vi "4461 - Create IO Channels Parallel.vi"(6 "error in":errorcluster, 7 "AI Buffer Size (S)":i32=10, 8 "sampling info":cluster{"Fs":dbl, "#s":dbl}, 9 "AO":T1={"AO amp (V)"=[0.1, 0.09, 0.08, 0.07, 0.06, 0.05, 0.04, 0.03], "AO DC (V)"=[0.0, 0.0, 0.0, 0.0, 0.0, 0.0, 0.0, 0.0], "AO f (Hz)"=[13.0, 13.0, 13.0, 13.0, 13.0, 13.0, 13.0, 13.0], "AO phi (deg)"=[0.0, 0.0, 0.0, 0.0, 0.0, 0.0, 0.0, 0.0], "function"=[enum."Sine Wave", enum."Sine Wave", enum."Sine Wave", enum."Sine Wave", enum."Sine Wave", enum."Sine Wave", enum."Sine Wave", enum."Sine Wave"]} {"AO DC (V)" format="%#_6p"; "AO amp (V)" format="%#_6p"}, 10 "AO Configuration":T2(array[cluster])=[{"Output physical channels"="PXI1Slot2/ao0", "AO. Max"=0.1, "AO.Min"=-0.1}, {"Output physical channels"="", "AO. Max"=0.1, "AO.Min"=-0.1}], 11 "AI Configuration":T3(array[cluster])=[{"AI.Coupling"=10050, "AI.Max"=10.0, "AI.Min"=-10.0, "Input physical channels"="PXI1Slot2/ai0:1"}, {"AI.Coupling"=10050, "AI.Max"=10.0, "AI.Min"=-10.0, "Input physical channels"="PXI1Slot3/ai0:3"}, {"AI.Coupling"=10050, "AI.Max"=10.0, "AI.Min"=-10.0, "Input physical channels"=""}] {"AI.Coupling" items=["AC"=10045, "DC"=10050, "GND"=10066]}) -> (2 "AO Task":refnum<k21>[](array[refnum]), 3 "AI task":refnum<k21>[](array[refnum]), 4 "error out":errorcluster, 5 "phase log":dbl[](array[numeric])=[0.99999999999938, 0.99999999999938])   [LabVIEW 2013]
uses:
  <vilib>/DAQmx/write.llb/DAQmx Write (Analog 1D Wfm NChan NSamp).vi
  <vilib>/DAQmx/create/channels.llb/DAQmx Create Channel (AO-Voltage-Basic).vi
  <vilib>/DAQmx/create/channels.llb/DAQmx Create Channel (AI-Voltage-Basic).vi
  <vilib>/DAQmx/configure/timing.llb/DAQmx Timing (Sample Clock).vi
  <vilib>/DAQmx/configure/trigger.llb/DAQmx Start Trigger (Digital Edge).vi
  <vilib>/DAQmx/miscellaneous.llb/DAQmx Fill In Error Info.vi
  <resource>/objmgr/daqmx.rc
panel:
  out "AI.FilterDelay":dbl
  out "AI.Gain":dbl
  in  "input terminal configuration":i32(ring)=-1 items=["default"=-1, "RSE"=10083, "NRSE"=10078, "Differential"=10106, "Pseudodifferential"=12529]
  in  "output terminal configuration":i32(ring)=-1 items=["Default"=-1, "RSE"=10083, "Differential"=10106, "Pseudodifferential"=12529]
  out "SampClk.Timebase.Rate":dbl
  out "SampQuant.SampPerChan":dbl
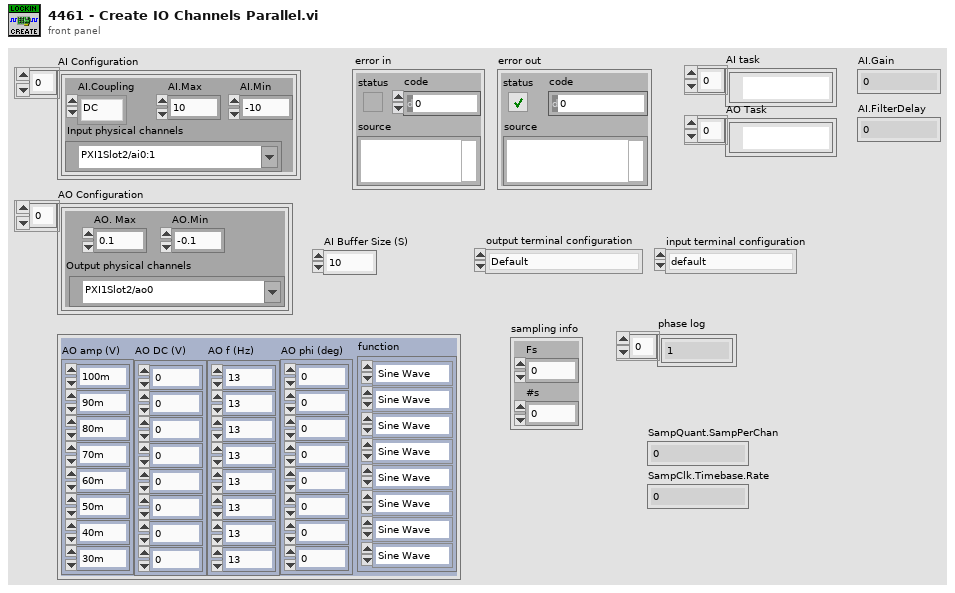
[diagram p1: front panel]
types:
  T1 = cluster{"AO amp (V)":dbl[], "AO DC (V)":dbl[], "AO f (Hz)":dbl[], "AO phi (deg)":dbl[], "function":enum16{"Sine Wave", "Triangle Wave", "Square Wave", "Sawtooth Wave"}[]}
  T2 = cluster{"Output physical channels":tag, "AO. Max":dbl, "AO.Min":dbl}[]
  T3 = cluster{"AI.Coupling":i32, "AI.Max":dbl, "AI.Min":dbl, "Input physical channels":tag}[]
  T4 = cluster{"AI.Coupling":i32, "AI.Max":dbl, "AI.Min":dbl, "Input physical channels":tag}
  T5 = cluster{"Output physical channels":tag, "AO. Max":dbl, "AO.Min":dbl}
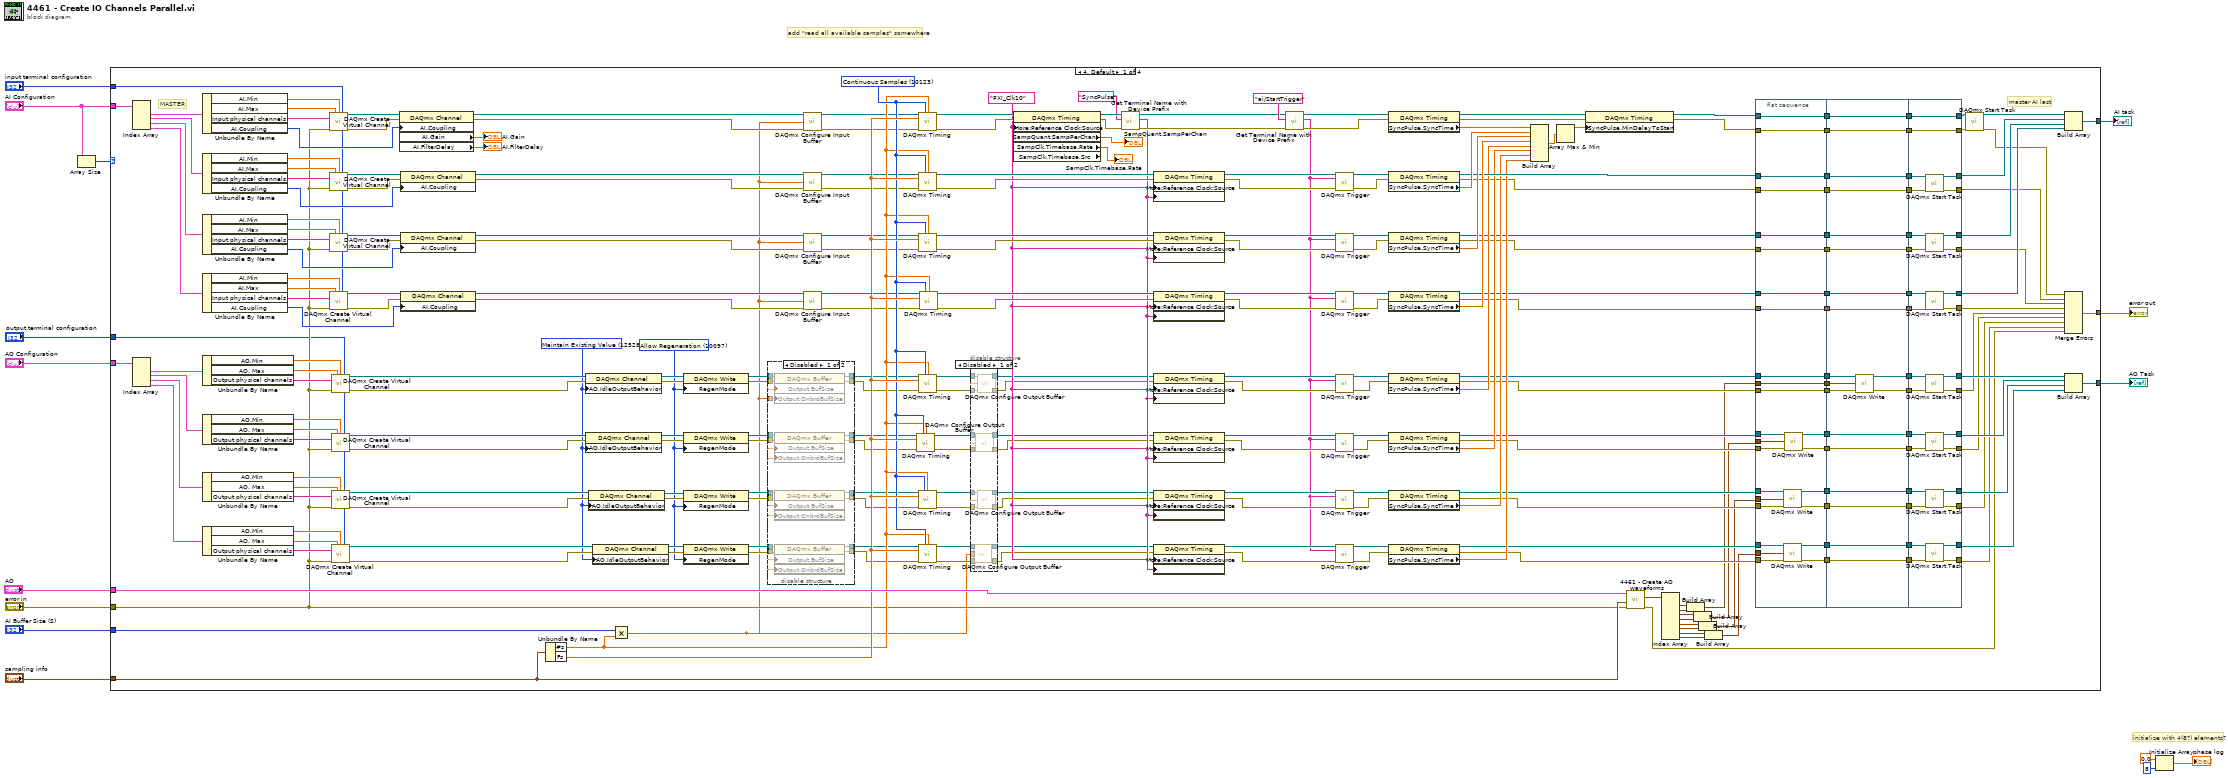
[diagram p0: block diagram]
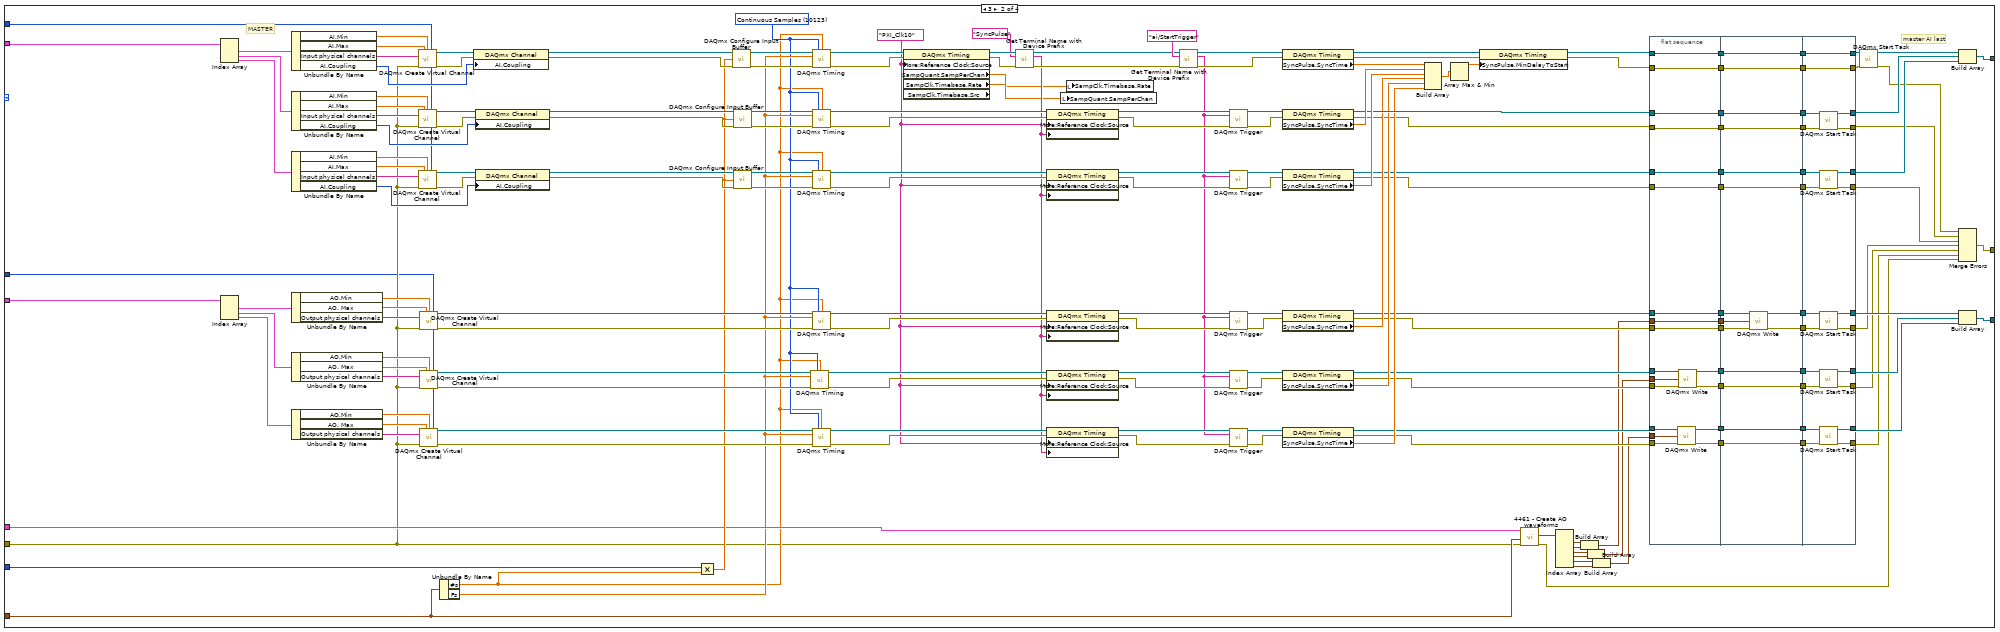
[diagram p4: hidden frame]
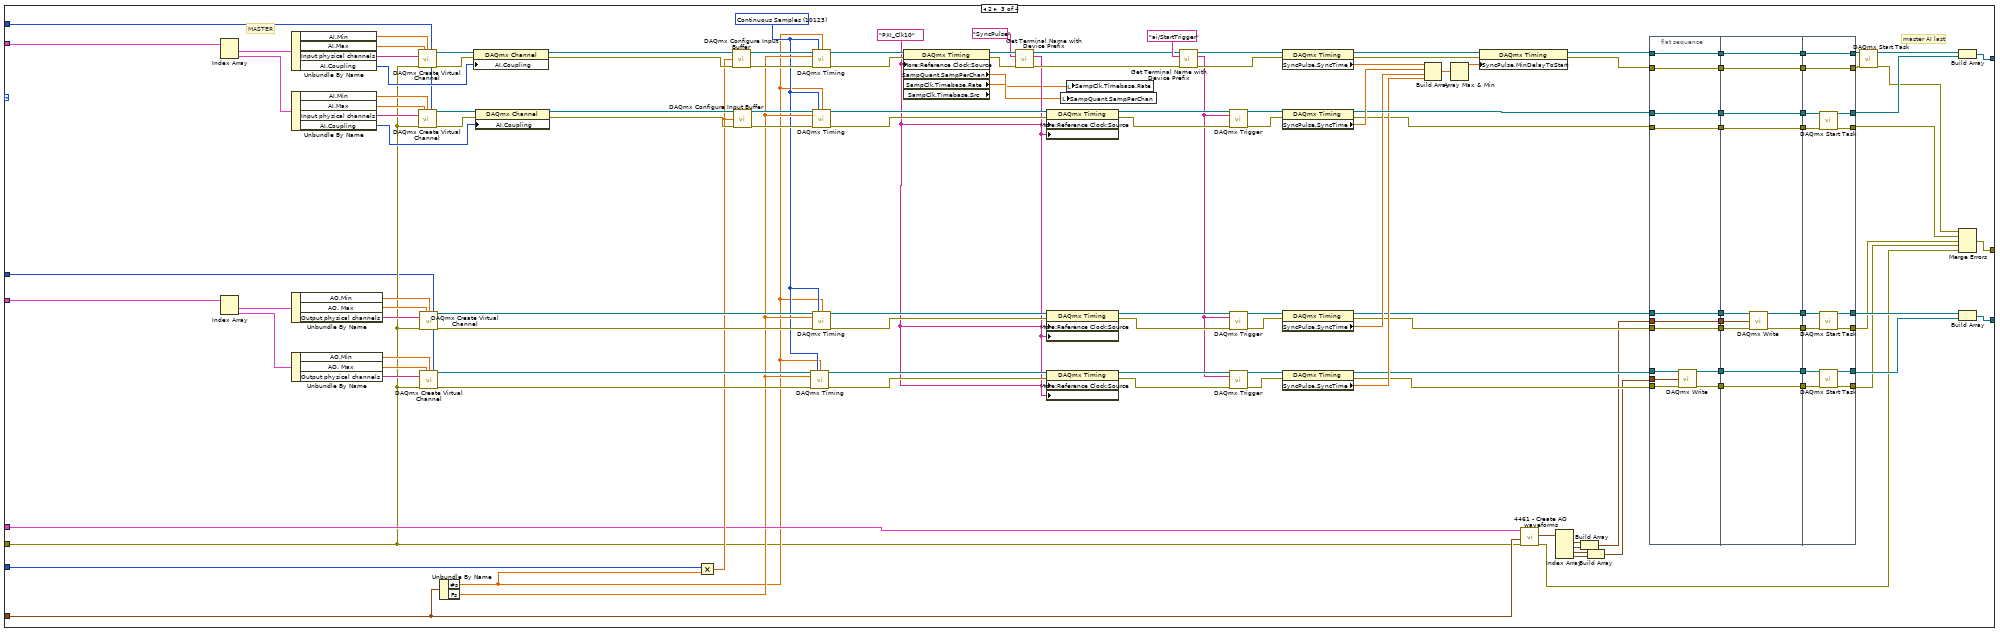
[diagram p5: hidden frame]
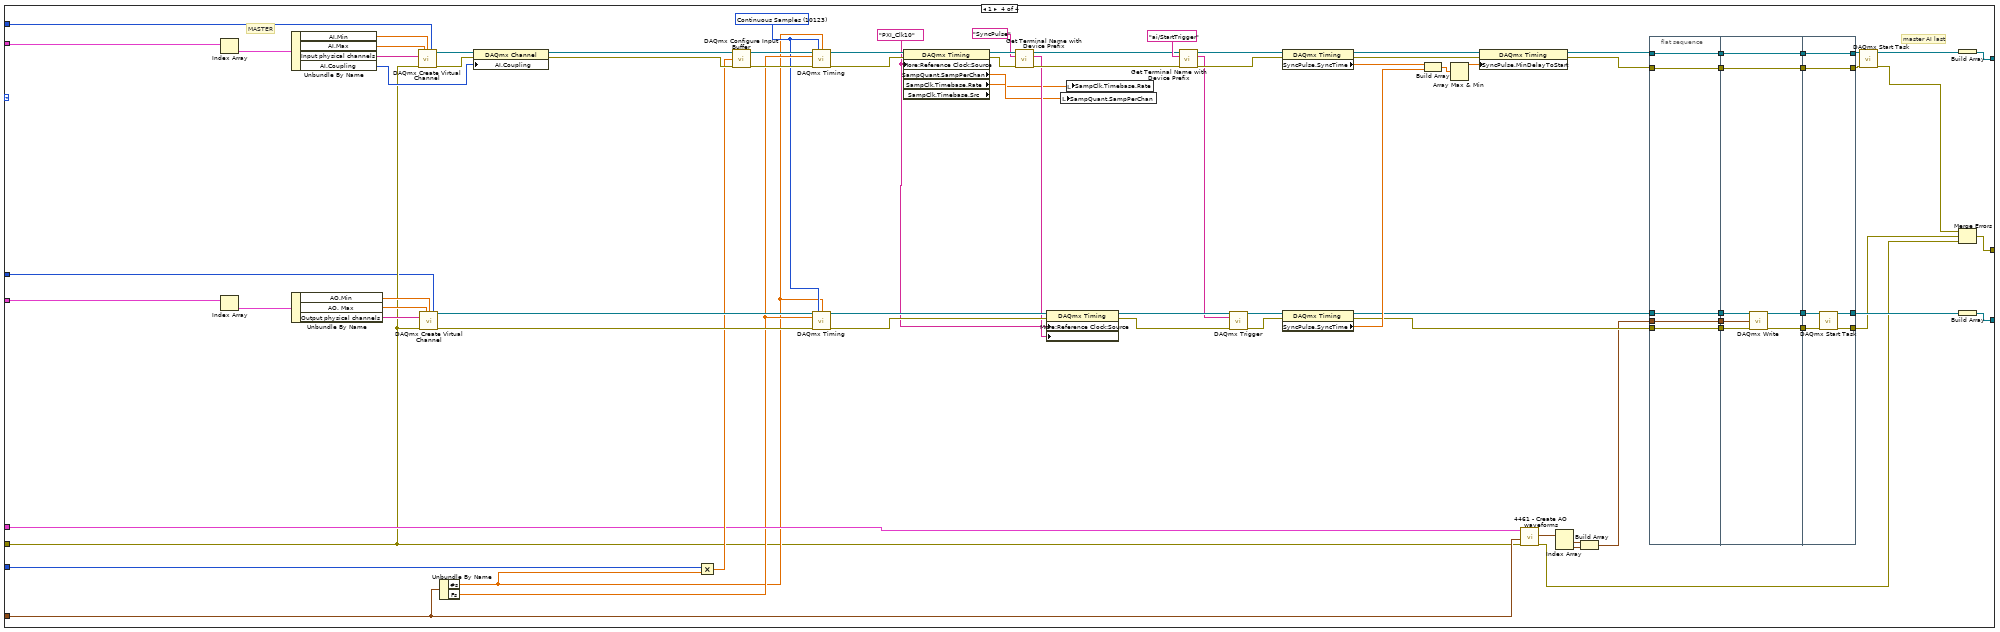
[diagram p6: hidden frame]
diagram:
  # "initialize with 4(8?) elements?"
  # "add \"read all available samples\" somewhere"
  n1 = Array Size(array="AI Configuration") -> (size(s)=w3:i32)
  n2 = case shown="4, Default" w3 {
    tunnel: "AI Buffer Size (S)" -> [w233 w545 w742 w870]
    tunnel: [w231 w543 w740 w868] -> w14
    tunnel: "AI Configuration" -> [w230 w542 w739 w867]
    tunnel: "AO Configuration" -> [w181 w499 w714 w861]
    tunnel: [w123 w446 w680 w845] -> w12
    tunnel: "AO" -> [w105 w428 w665 w833]
    tunnel: "sampling info" -> [w104 w427 w664 w832]
    tunnel: [w96 w420 w658 w827] -> w6
    tunnel: "error in" -> [w90 w415 w654 w824]
    tunnel: "output terminal configuration" -> [w85 w410 w650 w819]
    tunnel: "input terminal configuration" -> [w86 w411 w649 w820]
    frame 4, Default {
      w74 = 12528 items=["Zero Volts"=12526, "High-Impedance"=12527, "Maintain Existing Value"=12528] ("AO.IdleOutputBehavior")
      w49 = 10097 items=["Allow Regeneration"=10097, "Do Not Allow Regeneration"=10158] ("RegenMode")
      w118 = tag "PXI_Clk10" ("RefClk.Src")
      w102 = 10123 items=["Finite Samples"=10178, "Continuous Samples"=10123] ("sample mode")
      # "master AI last"
      # "MASTER"
      n3 = Index Array(array=w230) -> (element #1=w251:T4, element #2=w219:T4, element #3=w194:T4, element #4=w193:T4)  [unwired: 4 in]
      n4 = Index Array(array=w181) -> (element #1=w180:T5, element #2=w149:T5, element #3=w150:T5, element #4=w151:T5)  [unwired: 4 in]
      n5 = Unbundle By Name(w251) -> ("AI.Min"=w228:dbl, "AI.Max"=w229:dbl, "Input physical channels"=w236:tag, "AI.Coupling"=w227:i32)
      n6 = Unbundle By Name(w219) -> ("AI.Min"=w224:dbl, "AI.Max"=w223:dbl, "Input physical channels"=w220:tag, "AI.Coupling"=w225:i32)
      n7 = Unbundle By Name(w194) -> ("AI.Min"=w206:dbl, "AI.Max"=w207:dbl, "Input physical channels"=w210:tag, "AI.Coupling"=w205:i32)
      n8 = Unbundle By Name(w193) -> ("AI.Min"=w203:dbl, "AI.Max"=w202:dbl, "Input physical channels"=w199:tag, "AI.Coupling"=w204:i32)
      n9 = Unbundle By Name(w180) -> ("AO.Min"=w177:dbl, "AO. Max"=w178:dbl, "Output physical channels"=w179:tag)
      n10 = Unbundle By Name(w149) -> ("AO.Min"=w168:dbl, "AO. Max"=w167:dbl, "Output physical channels"=w166:tag)
      n11 = Unbundle By Name(w150) -> ("AO.Min"=w163:dbl, "AO. Max"=w164:dbl, "Output physical channels"=w165:tag)
      n12 = Unbundle By Name(w151) -> ("AO.Min"=w154:dbl, "AO. Max"=w153:dbl, "Output physical channels"=w152:tag)
      n13 = call-poly <vilib>:"DAQmx Create Virtual Channel.vi"("maximum value"=w229, "minimum value"=w228, "input terminal configuration"=w86, "physical channels"=w236, "error in"=w90) -> ("task out"=w235:refnum<k21>, "error out"=w234:errorcluster)  [unwired: 9 in]
      n14 = call-poly <vilib>:"DAQmx Create Virtual Channel.vi"("maximum value"=w223, "minimum value"=w224, "input terminal configuration"=w86, "physical channels"=w220, "error in"=w90) -> ("task out"=w221:refnum<k21>, "error out"=w222:errorcluster)  [unwired: 9 in]
      n15 = call-poly <vilib>:"DAQmx Create Virtual Channel.vi"("maximum value"=w207, "minimum value"=w206, "input terminal configuration"=w86, "physical channels"=w210, "error in"=w90) -> ("task out"=w209:refnum<k21>, "error out"=w208:errorcluster)  [unwired: 9 in]
      n16 = call-poly <vilib>:"DAQmx Create Virtual Channel.vi"("maximum value"=w202, "minimum value"=w203, "input terminal configuration"=w86, "physical channels"=w199, "error in"=w90) -> ("task out"=w200:refnum<k21>, "error out"=w201:errorcluster)  [unwired: 9 in]
      n17 = call-poly <vilib>:"DAQmx Create Virtual Channel.vi"("maximum value"=w178, "minimum value"=w177, "output terminal configuration"=w85, "physical channels"=w179, "error in"=w90) -> ("task out"=w82:refnum<k21>, "error out"=w81:errorcluster)  [unwired: 9 in]
      n18 = call-poly <vilib>:"DAQmx Create Virtual Channel.vi"("maximum value"=w167, "minimum value"=w168, "output terminal configuration"=w85, "physical channels"=w166, "error in"=w90) -> ("task out"=w75:refnum<k21>, "error out"=w76:errorcluster)  [unwired: 9 in]
      n19 = call-poly <vilib>:"DAQmx Create Virtual Channel.vi"("maximum value"=w164, "minimum value"=w163, "output terminal configuration"=w85, "physical channels"=w165, "error in"=w90) -> ("task out"=w77:refnum<k21>, "error out"=w78:errorcluster)  [unwired: 9 in]
      n20 = call-poly <vilib>:"DAQmx Create Virtual Channel.vi"("maximum value"=w153, "minimum value"=w154, "output terminal configuration"=w85, "physical channels"=w152, "error in"=w90) -> ("task out"=w80:refnum<k21>, "error out"=w79:errorcluster)  [unwired: 9 in]
      n21 = property class="DAQmx Channel"(reference=w235, error in=w234, "AI.Coupling"=w227) -> (reference out=w32:refnum<k21>, error out=w20:errorcluster, "AI.Gain"=→"AI.Gain":dbl, "AI.FilterDelay"=→"AI.FilterDelay":dbl)
      n22 = property class="DAQmx Channel"(reference=w221, error in=w222, "AI.Coupling"=w225) -> (reference out=w30:refnum<k21>, error out=w19:errorcluster)
      n23 = property class="DAQmx Channel"(reference=w209, error in=w208, "AI.Coupling"=w205) -> (reference out=w29:refnum<k21>, error out=w18:errorcluster)
      n24 = property class="DAQmx Channel"(reference=w200, error in=w201, "AI.Coupling"=w204) -> (reference out=w28:refnum<k21>, error out=w17:errorcluster)
      n25 = Unbundle By Name(w104) -> ("#s"=w101:dbl, "Fs"=w103:dbl)
      n26 = property class="DAQmx Channel"(reference=w82, error in=w81, "AO.IdleOutputBehavior"=w74) -> (reference out=w65:refnum<k21>, error out=w64:errorcluster)
      n27 = property class="DAQmx Channel"(reference=w75, error in=w76, "AO.IdleOutputBehavior"=w74) -> (reference out=w54:refnum<k21>, error out=w55:errorcluster)
      n28 = property class="DAQmx Channel"(reference=w77, error in=w78, "AO.IdleOutputBehavior"=w74) -> (reference out=w56:refnum<k21>, error out=w57:errorcluster)
      n29 = property class="DAQmx Channel"(reference=w80, error in=w79, "AO.IdleOutputBehavior"=w74) -> (reference out=w61:refnum<k21>, error out=w58:errorcluster)
      n30 = Multiply(x=w233, y=w101) -> (x*y=w16:dbl)
      n31 = property class="DAQmx Write"(reference=w65, error in=w64, "RegenMode"=w49) -> (reference out=w62:refnum<k21>, error out=w63:errorcluster)
      n32 = property class="DAQmx Write"(reference=w54, error in=w55, "RegenMode"=w49) -> (reference out=w53:refnum<k21>, error out=w52:errorcluster)
      n33 = property class="DAQmx Write"(reference=w56, error in=w57, "RegenMode"=w49) -> (reference out=w51:refnum<k21>, error out=w50:errorcluster)
      n34 = property class="DAQmx Write"(reference=w61, error in=w58, "RegenMode"=w49) -> (reference out=w60:refnum<k21>, error out=w59:errorcluster)
      n35 = disable-structure shown="Disabled" {
        disable-tunnel: [w326 w334] -> w73
        disable-tunnel: [w325 w332] -> w72
        disable-tunnel: [w324 w331] -> w71
        disable-tunnel: [w323 w333] -> w70
        disable-tunnel: [w322 w330] -> w69
        disable-tunnel: [w321 w329] -> w68
        disable-tunnel: [w320 w328] -> w67
        disable-tunnel: [w319 w327] -> w66
        disable-tunnel: w63 -> [w318 w333]
        disable-tunnel: w62 -> [w317 w334]
        disable-tunnel: w60 -> [w316 w328]
        disable-tunnel: w59 -> [w315 w327]
        disable-tunnel: w53 -> [w314 w332]
        disable-tunnel: w52 -> [w313 w331]
        disable-tunnel: w51 -> [w312 w330]
        disable-tunnel: w50 -> [w311 w329]
        disable-tunnel: w16 -> [w310 _]
        frame Disabled {
          n36 = property class="DAQmx Buffer"(reference=w317, error in=w318, "Output.BufSize"=w310, "Output.OnbrdBufSize"=w310) -> (reference out=w326:refnum<k21>, error out=w323:errorcluster)
          n37 = property class="DAQmx Buffer"(reference=w314, error in=w313, "Output.BufSize"=w310, "Output.OnbrdBufSize"=w310) -> (reference out=w325:refnum<k21>, error out=w324:errorcluster)
          n38 = property class="DAQmx Buffer"(reference=w312, error in=w311, "Output.BufSize"=w310, "Output.OnbrdBufSize"=w310) -> (reference out=w322:refnum<k21>, error out=w321:errorcluster)
          n39 = property class="DAQmx Buffer"(reference=w316, error in=w315, "Output.BufSize"=w310, "Output.OnbrdBufSize"=w310) -> (reference out=w320:refnum<k21>, error out=w319:errorcluster)
        }
        frame Enabled {
        }
      }
      n40 = call <vilib>:"DAQmx Configure Input Buffer.vi"("task/channels in"=w32, "buffer size (in samples per channel)"=w16, "error in"=w20) -> ("task out"=w31:refnum<k21>, "error out"=w21:errorcluster)  [unwired: 11 in]
      n41 = call <vilib>:"DAQmx Configure Input Buffer.vi"("task/channels in"=w30, "buffer size (in samples per channel)"=w16, "error in"=w19) -> ("task out"=w22:refnum<k21>, "error out"=w23:errorcluster)  [unwired: 11 in]
      n42 = call <vilib>:"DAQmx Configure Input Buffer.vi"("task/channels in"=w29, "buffer size (in samples per channel)"=w16, "error in"=w18) -> ("task out"=w26:refnum<k21>, "error out"=w25:errorcluster)  [unwired: 11 in]
      n43 = call <vilib>:"DAQmx Configure Input Buffer.vi"("task/channels in"=w28, "buffer size (in samples per channel)"=w16, "error in"=w17) -> ("task out"=w27:refnum<k21>, "error out"=w24:errorcluster)  [unwired: 11 in]
      n44 = call-poly <vilib>:"DAQmx Timing.vi"("task/channels in"=w72, "sample mode"=w102, "samples per channel"=w101, "rate"=w103, "error in"=w71) -> ("task out"=w48:refnum<k21>, "error out"=w47:errorcluster)  [unwired: 9 in]
      n45 = call-poly <vilib>:"DAQmx Timing.vi"("task/channels in"=w69, "sample mode"=w102, "samples per channel"=w101, "rate"=w103, "error in"=w68) -> ("task out"=w44:refnum<k21>, "error out"=w41:errorcluster)  [unwired: 9 in]
      n46 = call-poly <vilib>:"DAQmx Timing.vi"("task/channels in"=w31, "sample mode"=w102, "samples per channel"=w101, "rate"=w103, "error in"=w21) -> ("task out"=w250:refnum<k21>, "error out"=w226:errorcluster)  [unwired: 9 in]
      n47 = call-poly <vilib>:"DAQmx Timing.vi"("task/channels in"=w22, "sample mode"=w102, "samples per channel"=w101, "rate"=w103, "error in"=w23) -> ("task out"=w218:refnum<k21>, "error out"=w217:errorcluster)  [unwired: 9 in]
      n48 = call-poly <vilib>:"DAQmx Timing.vi"("task/channels in"=w26, "sample mode"=w102, "samples per channel"=w101, "rate"=w103, "error in"=w25) -> ("task out"=w211:refnum<k21>, "error out"=w212:errorcluster)  [unwired: 9 in]
      n49 = call-poly <vilib>:"DAQmx Timing.vi"("task/channels in"=w73, "sample mode"=w102, "samples per channel"=w101, "rate"=w103, "error in"=w70) -> ("task out"=w34:refnum<k21>, "error out"=w36:errorcluster)  [unwired: 9 in]
      n50 = call-poly <vilib>:"DAQmx Timing.vi"("task/channels in"=w67, "sample mode"=w102, "samples per channel"=w101, "rate"=w103, "error in"=w66) -> ("task out"=w43:refnum<k21>, "error out"=w42:errorcluster)  [unwired: 9 in]
      n51 = call-poly <vilib>:"DAQmx Timing.vi"("task/channels in"=w27, "sample mode"=w102, "samples per channel"=w101, "rate"=w103, "error in"=w24) -> ("task out"=w198:refnum<k21>, "error out"=w197:errorcluster)  [unwired: 9 in]
      n52 = disable-structure shown="Disabled" {
        disable-tunnel: w48 -> [w301 w304]
        disable-tunnel: w47 -> [w300 w305]
        disable-tunnel: [w299 w305] -> w46
        disable-tunnel: [w298 w304] -> w45
        disable-tunnel: w44 -> [w297 w306]
        disable-tunnel: w43 -> [w296 w308]
        disable-tunnel: w42 -> [w295 w309]
        disable-tunnel: w41 -> [w294 w307]
        disable-tunnel: [w293 w307] -> w40
        disable-tunnel: [w292 w309] -> w39
        disable-tunnel: [w291 w308] -> w38
        disable-tunnel: [w290 w306] -> w37
        disable-tunnel: w36 -> [w289 w303]
        disable-tunnel: [w288 w303] -> w35
        disable-tunnel: w34 -> [w287 w302]
        disable-tunnel: [w286 w302] -> w33
        disable-tunnel: w16 -> [w285 _]
        frame Disabled {
          n53 = call <vilib>:"DAQmx Configure Output Buffer.vi"("task/channels in"=w296, "buffer size (in samples per channel)"=w285, "error in"=w295) -> ("task out"=w291:refnum<k21>, "error out"=w292:errorcluster)  [unwired: 11 in]
          n54 = call <vilib>:"DAQmx Configure Output Buffer.vi"("task/channels in"=w301, "buffer size (in samples per channel)"=w285, "error in"=w300) -> ("task out"=w298:refnum<k21>, "error out"=w299:errorcluster)  [unwired: 11 in]
          n55 = call <vilib>:"DAQmx Configure Output Buffer.vi"("task/channels in"=w287, "buffer size (in samples per channel)"=w285, "error in"=w289) -> ("task out"=w286:refnum<k21>, "error out"=w288:errorcluster)  [unwired: 11 in]
          n56 = call <vilib>:"DAQmx Configure Output Buffer.vi"("task/channels in"=w297, "buffer size (in samples per channel)"=w285, "error in"=w294) -> ("task out"=w290:refnum<k21>, "error out"=w293:errorcluster)  [unwired: 11 in]
        }
        frame Enabled {
        }
      }
      n57 = property class="DAQmx Timing" props=["More:Reference Clock:Source", "SampQuant.SampPerChan", "SampClk.Timebase.Rate", "SampClk.Timebase.Src"](reference=w250, error in=w226, "More:Reference Clock:Source"=w118) -> (reference out=w122:refnum<k21>, error out=w121:errorcluster, "SampQuant.SampPerChan"=→"SampQuant.SampPerChan":dbl, "SampClk.Timebase.Rate"=→"SampClk.Timebase.Rate":dbl)  [unwired: 1 out]
      n58 = call "Get Terminal Name with Device Prefix.vi"("error in (no error)"=w121, "Local Terminal Name"="SyncPulse", "task/channels in"=w122) -> ("error out"=w245:errorcluster, "Terminal Name with Device Prefix"=w119:tag, "task out"=w246:refnum<k21>)  [unwired: 6 in]
      n59 = property class="DAQmx Timing"(reference=w218, error in=w217, "More:Reference Clock:Source"=w118, "More:Synchronization Pulse:Source"=w119) -> (reference out=w216:refnum<k21>, error out=w215:errorcluster)
      n60 = property class="DAQmx Timing"(reference=w211, error in=w212, "More:Reference Clock:Source"=w118, "More:Synchronization Pulse:Source"=w119) -> (reference out=w213:refnum<k21>, error out=w214:errorcluster)
      n61 = property class="DAQmx Timing"(reference=w198, error in=w197, "More:Reference Clock:Source"=w118, "More:Synchronization Pulse:Source"=w119) -> (reference out=w196:refnum<k21>, error out=w195:errorcluster)
      n62 = property class="DAQmx Timing"(reference=w33, error in=w35, "More:Reference Clock:Source"=w118, "More:Synchronization Pulse:Source"=w119) -> (reference out=w176:refnum<k21>, error out=w175:errorcluster)
      n63 = property class="DAQmx Timing"(reference=w45, error in=w46, "More:Reference Clock:Source"=w118, "More:Synchronization Pulse:Source"=w119) -> (reference out=w169:refnum<k21>, error out=w170:errorcluster)
      n64 = property class="DAQmx Timing"(reference=w37, error in=w40, "More:Reference Clock:Source"=w118, "More:Synchronization Pulse:Source"=w119) -> (reference out=w162:refnum<k21>, error out=w161:errorcluster)
      n65 = property class="DAQmx Timing"(reference=w38, error in=w39, "More:Reference Clock:Source"=w118, "More:Synchronization Pulse:Source"=w119) -> (reference out=w155:refnum<k21>, error out=w156:errorcluster)
      n66 = call "Get Terminal Name with Device Prefix.vi"("error in (no error)"=w245, "Local Terminal Name"="ai/StartTrigger", "task/channels in"=w246) -> ("error out"=w243:errorcluster, "Terminal Name with Device Prefix"=w144:tag, "task out"=w244:refnum<k21>)  [unwired: 6 in]
      n67 = call-poly <vilib>:"DAQmx Trigger.vi"("task/channels in"=w216, "source"=w144, "error in"=w215) -> ("task out"=w190:refnum<k21>, "error out"=w189:errorcluster)  [unwired: 11 in]
      n68 = call-poly <vilib>:"DAQmx Trigger.vi"("task/channels in"=w213, "source"=w144, "error in"=w214) -> ("task out"=w191:refnum<k21>, "error out"=w188:errorcluster)  [unwired: 11 in]
      n69 = call-poly <vilib>:"DAQmx Trigger.vi"("task/channels in"=w196, "source"=w144, "error in"=w195) -> ("task out"=w192:refnum<k21>, "error out"=w187:errorcluster)  [unwired: 11 in]
      n70 = call-poly <vilib>:"DAQmx Trigger.vi"("task/channels in"=w176, "source"=w144, "error in"=w175) -> ("task out"=w174:refnum<k21>, "error out"=w173:errorcluster)  [unwired: 11 in]
      n71 = call-poly <vilib>:"DAQmx Trigger.vi"("task/channels in"=w169, "source"=w144, "error in"=w170) -> ("task out"=w171:refnum<k21>, "error out"=w172:errorcluster)  [unwired: 11 in]
      n72 = call-poly <vilib>:"DAQmx Trigger.vi"("task/channels in"=w162, "source"=w144, "error in"=w161) -> ("task out"=w160:refnum<k21>, "error out"=w159:errorcluster)  [unwired: 11 in]
      n73 = call-poly <vilib>:"DAQmx Trigger.vi"("task/channels in"=w155, "source"=w144, "error in"=w156) -> ("task out"=w157:refnum<k21>, "error out"=w158:errorcluster)  [unwired: 11 in]
      n74 = property class="DAQmx Timing"(reference=w244, error in=w243) -> (reference out=w240:refnum<k21>, error out=w241:errorcluster, "SyncPulse.SyncTime"=w242:dbl)
      n75 = property class="DAQmx Timing"(reference=w190, error in=w189) -> (reference out=w182:refnum<k21>, error out=w141:errorcluster, "SyncPulse.SyncTime"=w185:dbl)
      n76 = property class="DAQmx Timing"(reference=w191, error in=w188) -> (reference out=w143:refnum<k21>, error out=w140:errorcluster, "SyncPulse.SyncTime"=w184:dbl)
      n77 = property class="DAQmx Timing"(reference=w192, error in=w187) -> (reference out=w142:refnum<k21>, error out=w139:errorcluster, "SyncPulse.SyncTime"=w183:dbl)
      n78 = property class="DAQmx Timing"(reference=w174, error in=w173) -> (reference out=w138:refnum<k21>, error out=w135:errorcluster, "SyncPulse.SyncTime"=w148:dbl)
      n79 = property class="DAQmx Timing"(reference=w171, error in=w172) -> (reference out=w137:refnum<k21>, error out=w134:errorcluster, "SyncPulse.SyncTime"=w147:dbl)
      n80 = property class="DAQmx Timing"(reference=w160, error in=w159) -> (reference out=w136:refnum<k21>, error out=w133:errorcluster, "SyncPulse.SyncTime"=w146:dbl)
      n81 = property class="DAQmx Timing"(reference=w157, error in=w158) -> (reference out=w132:refnum<k21>, error out=w131:errorcluster, "SyncPulse.SyncTime"=w145:dbl)
      n82 = Build Array(w242, w185, w184, w183, w148, w147, w146, w145) -> (w239:dbl[])
      n83 = Array Max & Min(array=w239) -> (max value=w186:dbl)  [unwired: 3 out]
      n84 = property class="DAQmx Timing"(reference=w240, error in=w241, "SyncPulse.MinDelayToStart"=w186) -> (reference out=w237:refnum<k21>, error out=w238:errorcluster)
      n85 = call "4461 - Create AO waveforms.vi"("error in (no error)"=w90, "sampling info"=w104, "AO"=w105) -> ("error out"=w89:errorcluster, "AO Array"=w91:waveform(dbl)[])  [unwired: 5 in, 2 out]
      n86 = Index Array(array=w91) -> (element #1=w106:waveform(dbl), element #2=w117:waveform(dbl), element #3=w116:waveform(dbl), element #4=w115:waveform(dbl), element #5=w114:waveform(dbl), element #6=w113:waveform(dbl), element #7=w112:waveform(dbl), element #8=w111:waveform(dbl))  [unwired: 8 in]
      n87 = Build Array(w106, w117) -> (w110:waveform(dbl)[])
      n88 = Build Array(w116, w115) -> (w109:waveform(dbl)[])
      n89 = Build Array(w114, w113) -> (w108:waveform(dbl)[])
      n90 = Build Array(w112, w111) -> (w107:waveform(dbl)[])
      n91 = flat-sequence {
        tunnel: w238 -> [w359]
        tunnel: w237 -> [w360]
        tunnel: [w360] -> w284
        tunnel: [w359] -> w283
        tunnel: [w358] -> w282
        tunnel: w182 -> [w358]
        tunnel: [w357] -> w281
        tunnel: w143 -> [w357]
        tunnel: [w356] -> w280
        tunnel: w142 -> [w356]
        tunnel: [w355] -> w279
        tunnel: w141 -> [w355]
        tunnel: [w354] -> w278
        tunnel: w140 -> [w354]
        tunnel: [w353] -> w277
        tunnel: w139 -> [w353]
        tunnel: [w352] -> w276
        tunnel: w138 -> [w352]
        tunnel: [w340] -> w275
        tunnel: w137 -> [w341]
        tunnel: [w344] -> w274
        tunnel: w136 -> [w343]
        tunnel: [w351] -> w273
        tunnel: w135 -> [w351]
        tunnel: w134 -> [w342]
        tunnel: [w345] -> w272
        tunnel: w133 -> [w346]
        tunnel: [w347] -> w271
        tunnel: w132 -> [w350]
        tunnel: [w348] -> w270
        tunnel: w131 -> [w349]
        tunnel: [w339] -> w269
        tunnel: [w338] -> w268
        tunnel: w110 -> [w338]
        tunnel: w109 -> [w337]
        tunnel: w108 -> [w336]
        tunnel: w107 -> [w335]
        tunnel: [w379] -> w267
        tunnel: [w378] -> w266
        tunnel: w284 -> [w379]
        tunnel: w283 -> [w378]
        tunnel: [w377] -> w265
        tunnel: w282 -> [w377]
        tunnel: [w376] -> w264
        tunnel: w281 -> [w376]
        tunnel: [w375] -> w263
        tunnel: w280 -> [w375]
        tunnel: [w374] -> w262
        tunnel: w279 -> [w374]
        tunnel: [w373] -> w261
        tunnel: w278 -> [w373]
        tunnel: [w372] -> w260
        tunnel: w277 -> [w372]
        tunnel: [w364] -> w259
        tunnel: w276 -> [w365]
        tunnel: [w371] -> w258
        tunnel: w275 -> [w371]
        tunnel: [w370] -> w257
        tunnel: w274 -> [w370]
        tunnel: [w363] -> w256
        tunnel: w273 -> [w362]
        tunnel: [w369] -> w255
        tunnel: [w368] -> w254
        tunnel: w272 -> [w368]
        tunnel: [w367] -> w253
        tunnel: w271 -> [w367]
        tunnel: [w366] -> w252
        tunnel: w270 -> [w366]
        tunnel: w269 -> [w369]
        tunnel: w268 -> [w361]
        tunnel: [w409] -> w249
        tunnel: [w408] -> w248
        tunnel: w267 -> [w409]
        tunnel: w266 -> [w408]
        tunnel: w265 -> [w407]
        tunnel: w264 -> [w406]
        tunnel: w263 -> [w405]
        tunnel: w262 -> [w404]
        tunnel: w261 -> [w403]
        tunnel: w260 -> [w402]
        tunnel: w259 -> [w401]
        tunnel: w258 -> [w400]
        tunnel: w257 -> [w399]
        tunnel: w256 -> [w398]
        tunnel: w255 -> [w397]
        tunnel: w254 -> [w396]
        tunnel: w253 -> [w395]
        tunnel: w252 -> [w394]
        tunnel: [w393] -> w130
        tunnel: [w392] -> w129
        tunnel: [w391] -> w128
        tunnel: [w390] -> w127
        tunnel: [w389] -> w126
        tunnel: [w388] -> w125
        tunnel: [w387] -> w124
        tunnel: [w386] -> w99
        tunnel: [w385] -> w98
        tunnel: [w384] -> w97
        tunnel: [w383] -> w95
        tunnel: [w382] -> w94
        tunnel: [w381] -> w93
        tunnel: [w380] -> w92
        frame #0 {
          n92 = call-poly <vilib>:"DAQmx Write.vi"("task/channels in"=w343, "data"=w336, "error in"=w346) -> ("task out"=w344:refnum<k21>, "error out"=w345:errorcluster)  [unwired: 10 in, 1 out]
          n93 = call-poly <vilib>:"DAQmx Write.vi"("task/channels in"=w350, "data"=w335, "error in"=w349) -> ("task out"=w347:refnum<k21>, "error out"=w348:errorcluster)  [unwired: 10 in, 1 out]
          n94 = call-poly <vilib>:"DAQmx Write.vi"("task/channels in"=w341, "data"=w337, "error in"=w342) -> ("task out"=w340:refnum<k21>, "error out"=w339:errorcluster)  [unwired: 10 in, 1 out]
        }
        frame #1 {
          n95 = call-poly <vilib>:"DAQmx Write.vi"("task/channels in"=w365, "data"=w361, "error in"=w362) -> ("task out"=w364:refnum<k21>, "error out"=w363:errorcluster)  [unwired: 10 in, 1 out]
        }
        frame #2 {
          n96 = call <vilib>:"DAQmx Start Task.vi"("task/channels in"=w407, "error in"=w404) -> ("task out"=w393:refnum<k21>, "error out"=w386:errorcluster)  [unwired: 12 in]
          n97 = call <vilib>:"DAQmx Start Task.vi"("task/channels in"=w406, "error in"=w403) -> ("task out"=w392:refnum<k21>, "error out"=w385:errorcluster)  [unwired: 12 in]
          n98 = call <vilib>:"DAQmx Start Task.vi"("task/channels in"=w405, "error in"=w402) -> ("task out"=w391:refnum<k21>, "error out"=w384:errorcluster)  [unwired: 12 in]
          n99 = call <vilib>:"DAQmx Start Task.vi"("task/channels in"=w401, "error in"=w398) -> ("task out"=w390:refnum<k21>, "error out"=w383:errorcluster)  [unwired: 12 in]
          n100 = call <vilib>:"DAQmx Start Task.vi"("task/channels in"=w400, "error in"=w397) -> ("task out"=w389:refnum<k21>, "error out"=w382:errorcluster)  [unwired: 12 in]
          n101 = call <vilib>:"DAQmx Start Task.vi"("task/channels in"=w399, "error in"=w396) -> ("task out"=w388:refnum<k21>, "error out"=w381:errorcluster)  [unwired: 12 in]
          n102 = call <vilib>:"DAQmx Start Task.vi"("task/channels in"=w395, "error in"=w394) -> ("task out"=w387:refnum<k21>, "error out"=w380:errorcluster)  [unwired: 12 in]
        }
      }
      n103 = call <vilib>:"DAQmx Start Task.vi"("task/channels in"=w249, "error in"=w248) -> ("task out"=w232:refnum<k21>, "error out"=w100:errorcluster)  [unwired: 12 in]
      n104 = Build Array(w232, w130, w129, w128) -> (w231:refnum<k21>[])
      n105 = Merge Errors(w100, w99, w98, w97, w95, w94, w93, w92, w89) -> (w96:errorcluster)
      n106 = Build Array(w127, w126, w125, w124) -> (w123:refnum<k21>[])
    }
    frame 3 {
      w441 = tag "PXI_Clk10" ("RefClk.Src")
      w425 = 10123 items=["Finite Samples"=10178, "Continuous Samples"=10123] ("sample mode")
      # "master AI last"
      # "MASTER"
      n107 = Index Array(array=w542) -> (element #1=w567:T4, element #2=w529:T4, element #3=w508:T4)  [unwired: 3 in]
      n108 = Index Array(array=w499) -> (element #1=w498:T5, element #2=w465:T5, element #3=w466:T5)  [unwired: 3 in]
      n109 = Unbundle By Name(w567) -> ("AI.Min"=w540:dbl, "AI.Max"=w541:dbl, "Input physical channels"=w552:tag, "AI.Coupling"=w539:i32)
      n110 = Unbundle By Name(w529) -> ("AI.Min"=w536:dbl, "AI.Max"=w535:dbl, "Input physical channels"=w530:tag, "AI.Coupling"=w537:i32)
      n111 = Unbundle By Name(w508) -> ("AI.Min"=w510:dbl, "AI.Max"=w511:dbl, "Input physical channels"=w516:tag, "AI.Coupling"=w509:i32)
      n112 = Unbundle By Name(w498) -> ("AO.Min"=w495:dbl, "AO. Max"=w496:dbl, "Output physical channels"=w497:tag)
      n113 = Unbundle By Name(w465) -> ("AO.Min"=w480:dbl, "AO. Max"=w479:dbl, "Output physical channels"=w478:tag)
      n114 = Unbundle By Name(w466) -> ("AO.Min"=w475:dbl, "AO. Max"=w476:dbl, "Output physical channels"=w477:tag)
      n115 = call-poly <vilib>:"DAQmx Create Virtual Channel.vi"("maximum value"=w541, "minimum value"=w540, "input terminal configuration"=w411, "physical channels"=w552, "error in"=w415) -> ("task out"=w551:refnum<k21>, "error out"=w550:errorcluster)  [unwired: 9 in]
      n116 = call-poly <vilib>:"DAQmx Create Virtual Channel.vi"("maximum value"=w535, "minimum value"=w536, "input terminal configuration"=w411, "physical channels"=w530, "error in"=w415) -> ("task out"=w531:refnum<k21>, "error out"=w532:errorcluster)  [unwired: 9 in]
      n117 = call-poly <vilib>:"DAQmx Create Virtual Channel.vi"("maximum value"=w511, "minimum value"=w510, "input terminal configuration"=w411, "physical channels"=w516, "error in"=w415) -> ("task out"=w515:refnum<k21>, "error out"=w514:errorcluster)  [unwired: 9 in]
      n118 = call-poly <vilib>:"DAQmx Create Virtual Channel.vi"("maximum value"=w496, "minimum value"=w495, "output terminal configuration"=w410, "physical channels"=w497, "error in"=w415) -> ("task out"=w440:refnum<k21>, "error out"=w439:errorcluster)  [unwired: 9 in]
      n119 = call-poly <vilib>:"DAQmx Create Virtual Channel.vi"("maximum value"=w479, "minimum value"=w480, "output terminal configuration"=w410, "physical channels"=w478, "error in"=w415) -> ("task out"=w481:refnum<k21>, "error out"=w482:errorcluster)  [unwired: 9 in]
      n120 = call-poly <vilib>:"DAQmx Create Virtual Channel.vi"("maximum value"=w476, "minimum value"=w475, "output terminal configuration"=w410, "physical channels"=w477, "error in"=w415) -> ("task out"=w474:refnum<k21>, "error out"=w473:errorcluster)  [unwired: 9 in]
      n121 = Unbundle By Name(w427) -> ("#s"=w424:dbl, "Fs"=w426:dbl)
      n122 = property class="DAQmx Channel"(reference=w551, error in=w550, "AI.Coupling"=w539) -> (reference out=w549:refnum<k21>, error out=w548:errorcluster)
      n123 = property class="DAQmx Channel"(reference=w531, error in=w532, "AI.Coupling"=w537) -> (reference out=w533:refnum<k21>, error out=w534:errorcluster)
      n124 = property class="DAQmx Channel"(reference=w515, error in=w514, "AI.Coupling"=w509) -> (reference out=w513:refnum<k21>, error out=w512:errorcluster)
      n125 = Multiply(x=w545, y=w424) -> (x*y=w429:dbl)
      n126 = call <vilib>:"DAQmx Configure Input Buffer.vi"("task/channels in"=w549, "buffer size (in samples per channel)"=w429, "error in"=w548) -> ("task out"=w547:refnum<k21>, "error out"=w546:errorcluster)  [unwired: 11 in]
      n127 = call <vilib>:"DAQmx Configure Input Buffer.vi"("task/channels in"=w533, "buffer size (in samples per channel)"=w429, "error in"=w534) -> ("task out"=w528:refnum<k21>, "error out"=w527:errorcluster)  [unwired: 11 in]
      n128 = call <vilib>:"DAQmx Configure Input Buffer.vi"("task/channels in"=w513, "buffer size (in samples per channel)"=w429, "error in"=w512) -> ("task out"=w517:refnum<k21>, "error out"=w518:errorcluster)  [unwired: 11 in]
      n129 = call-poly <vilib>:"DAQmx Timing.vi"("task/channels in"=w481, "sample mode"=w425, "samples per channel"=w424, "rate"=w426, "error in"=w482) -> ("task out"=w484:refnum<k21>, "error out"=w485:errorcluster)  [unwired: 9 in]
      n130 = call-poly <vilib>:"DAQmx Timing.vi"("task/channels in"=w474, "sample mode"=w425, "samples per channel"=w424, "rate"=w426, "error in"=w473) -> ("task out"=w471:refnum<k21>, "error out"=w470:errorcluster)  [unwired: 9 in]
      n131 = call-poly <vilib>:"DAQmx Timing.vi"("task/channels in"=w547, "sample mode"=w425, "samples per channel"=w424, "rate"=w426, "error in"=w546) -> ("task out"=w566:refnum<k21>, "error out"=w538:errorcluster)  [unwired: 9 in]
      n132 = call-poly <vilib>:"DAQmx Timing.vi"("task/channels in"=w528, "sample mode"=w425, "samples per channel"=w424, "rate"=w426, "error in"=w527) -> ("task out"=w526:refnum<k21>, "error out"=w525:errorcluster)  [unwired: 9 in]
      n133 = call-poly <vilib>:"DAQmx Timing.vi"("task/channels in"=w517, "sample mode"=w425, "samples per channel"=w424, "rate"=w426, "error in"=w518) -> ("task out"=w519:refnum<k21>, "error out"=w520:errorcluster)  [unwired: 9 in]
      n134 = call-poly <vilib>:"DAQmx Timing.vi"("task/channels in"=w440, "sample mode"=w425, "samples per channel"=w424, "rate"=w426, "error in"=w439) -> ("task out"=w493:refnum<k21>, "error out"=w492:errorcluster)  [unwired: 9 in]
      n135 = property class="DAQmx Timing" props=["More:Reference Clock:Source", "SampQuant.SampPerChan", "SampClk.Timebase.Rate", "SampClk.Timebase.Src"](reference=w566, error in=w538, "More:Reference Clock:Source"=w441) -> (reference out=w445:refnum<k21>, error out=w444:errorcluster, "SampQuant.SampPerChan"=w413:dbl, "SampClk.Timebase.Rate"=w412:dbl)  [unwired: 1 out]
      n136 = call "Get Terminal Name with Device Prefix.vi"("error in (no error)"=w444, "Local Terminal Name"="SyncPulse", "task/channels in"=w445) -> ("error out"=w561:errorcluster, "Terminal Name with Device Prefix"=w442:tag, "task out"=w562:refnum<k21>)  [unwired: 6 in]
      n137 = property class="DAQmx Timing"(reference=w526, error in=w525, "More:Reference Clock:Source"=w441, "More:Synchronization Pulse:Source"=w442) -> (reference out=w524:refnum<k21>, error out=w523:errorcluster)
      n138 = property class="DAQmx Timing"(reference=w519, error in=w520, "More:Reference Clock:Source"=w441, "More:Synchronization Pulse:Source"=w442) -> (reference out=w521:refnum<k21>, error out=w522:errorcluster)
      n139 = property class="DAQmx Timing"(reference=w493, error in=w492, "More:Reference Clock:Source"=w441, "More:Synchronization Pulse:Source"=w442) -> (reference out=w494:refnum<k21>, error out=w491:errorcluster)
      n140 = property class="DAQmx Timing"(reference=w484, error in=w485, "More:Reference Clock:Source"=w441, "More:Synchronization Pulse:Source"=w442) -> (reference out=w483:refnum<k21>, error out=w486:errorcluster)
      n141 = property class="DAQmx Timing"(reference=w471, error in=w470, "More:Reference Clock:Source"=w441, "More:Synchronization Pulse:Source"=w442) -> (reference out=w472:refnum<k21>, error out=w469:errorcluster)
      n142 = local write "SampQuant.SampPerChan"(w413) -> ()
      n143 = local write "SampClk.Timebase.Rate"(w412) -> ()
      n144 = call "Get Terminal Name with Device Prefix.vi"("error in (no error)"=w561, "Local Terminal Name"="ai/StartTrigger", "task/channels in"=w562) -> ("error out"=w559:errorcluster, "Terminal Name with Device Prefix"=w461:tag, "task out"=w560:refnum<k21>)  [unwired: 6 in]
      n145 = call-poly <vilib>:"DAQmx Trigger.vi"("task/channels in"=w524, "source"=w461, "error in"=w523) -> ("task out"=w506:refnum<k21>, "error out"=w505:errorcluster)  [unwired: 11 in]
      n146 = call-poly <vilib>:"DAQmx Trigger.vi"("task/channels in"=w521, "source"=w461, "error in"=w522) -> ("task out"=w507:refnum<k21>, "error out"=w504:errorcluster)  [unwired: 11 in]
      n147 = call-poly <vilib>:"DAQmx Trigger.vi"("task/channels in"=w494, "source"=w461, "error in"=w491) -> ("task out"=w490:refnum<k21>, "error out"=w489:errorcluster)  [unwired: 11 in]
      n148 = call-poly <vilib>:"DAQmx Trigger.vi"("task/channels in"=w483, "source"=w461, "error in"=w486) -> ("task out"=w487:refnum<k21>, "error out"=w488:errorcluster)  [unwired: 11 in]
      n149 = call-poly <vilib>:"DAQmx Trigger.vi"("task/channels in"=w472, "source"=w461, "error in"=w469) -> ("task out"=w468:refnum<k21>, "error out"=w467:errorcluster)  [unwired: 11 in]
      n150 = property class="DAQmx Timing"(reference=w560, error in=w559) -> (reference out=w556:refnum<k21>, error out=w557:errorcluster, "SyncPulse.SyncTime"=w558:dbl)
      n151 = property class="DAQmx Timing"(reference=w506, error in=w505) -> (reference out=w500:refnum<k21>, error out=w459:errorcluster, "SyncPulse.SyncTime"=w502:dbl)
      n152 = property class="DAQmx Timing"(reference=w507, error in=w504) -> (reference out=w460:refnum<k21>, error out=w458:errorcluster, "SyncPulse.SyncTime"=w501:dbl)
      n153 = property class="DAQmx Timing"(reference=w490, error in=w489) -> (reference out=w457:refnum<k21>, error out=w454:errorcluster, "SyncPulse.SyncTime"=w464:dbl)
      n154 = property class="DAQmx Timing"(reference=w487, error in=w488) -> (reference out=w456:refnum<k21>, error out=w453:errorcluster, "SyncPulse.SyncTime"=w463:dbl)
      n155 = property class="DAQmx Timing"(reference=w468, error in=w467) -> (reference out=w455:refnum<k21>, error out=w452:errorcluster, "SyncPulse.SyncTime"=w462:dbl)
      n156 = Build Array(w558, w502, w501, w464, w463, w462) -> (w555:dbl[])
      n157 = Array Max & Min(array=w555) -> (max value=w503:dbl)  [unwired: 3 out]
      n158 = property class="DAQmx Timing"(reference=w556, error in=w557, "SyncPulse.MinDelayToStart"=w503) -> (reference out=w553:refnum<k21>, error out=w554:errorcluster)
      n159 = call "4461 - Create AO waveforms.vi"("error in (no error)"=w415, "sampling info"=w427, "AO"=w428) -> ("error out"=w414:errorcluster, "AO Array"=w416:waveform(dbl)[])  [unwired: 5 in, 2 out]
      n160 = Index Array(array=w416) -> (element #1=w430:waveform(dbl), element #2=w438:waveform(dbl), element #3=w437:waveform(dbl), element #4=w436:waveform(dbl), element #5=w435:waveform(dbl), element #6=w434:waveform(dbl))  [unwired: 6 in]
      n161 = Build Array(w430, w438) -> (w433:waveform(dbl)[])
      n162 = Build Array(w437, w436) -> (w432:waveform(dbl)[])
      n163 = Build Array(w435, w434) -> (w431:waveform(dbl)[])
      n164 = flat-sequence {
        tunnel: w554 -> [w610]
        tunnel: w553 -> [w611]
        tunnel: [w611] -> w592
        tunnel: [w610] -> w591
        tunnel: [w609] -> w590
        tunnel: w500 -> [w609]
        tunnel: [w608] -> w589
        tunnel: w460 -> [w608]
        tunnel: [w607] -> w588
        tunnel: w459 -> [w607]
        tunnel: [w606] -> w587
        tunnel: w458 -> [w606]
        tunnel: [w605] -> w586
        tunnel: w457 -> [w605]
        tunnel: [w597] -> w585
        tunnel: w456 -> [w598]
        tunnel: [w601] -> w584
        tunnel: w455 -> [w600]
        tunnel: [w604] -> w583
        tunnel: w454 -> [w604]
        tunnel: w453 -> [w599]
        tunnel: [w602] -> w582
        tunnel: w452 -> [w603]
        tunnel: [w596] -> w581
        tunnel: [w595] -> w580
        tunnel: w433 -> [w595]
        tunnel: w432 -> [w594]
        tunnel: w431 -> [w593]
        tunnel: [w626] -> w579
        tunnel: [w625] -> w578
        tunnel: w592 -> [w626]
        tunnel: w591 -> [w625]
        tunnel: [w624] -> w577
        tunnel: w590 -> [w624]
        tunnel: [w623] -> w576
        tunnel: w589 -> [w623]
        tunnel: [w622] -> w575
        tunnel: w588 -> [w622]
        tunnel: [w621] -> w574
        tunnel: w587 -> [w621]
        tunnel: [w615] -> w573
        tunnel: w586 -> [w616]
        tunnel: [w620] -> w572
        tunnel: w585 -> [w620]
        tunnel: [w619] -> w571
        tunnel: w584 -> [w619]
        tunnel: [w614] -> w570
        tunnel: w583 -> [w613]
        tunnel: [w618] -> w569
        tunnel: [w617] -> w568
        tunnel: w582 -> [w617]
        tunnel: w581 -> [w618]
        tunnel: w580 -> [w612]
        tunnel: [w648] -> w565
        tunnel: [w647] -> w564
        tunnel: w579 -> [w648]
        tunnel: w578 -> [w647]
        tunnel: w577 -> [w646]
        tunnel: w576 -> [w645]
        tunnel: w575 -> [w644]
        tunnel: w574 -> [w643]
        tunnel: w573 -> [w642]
        tunnel: w572 -> [w641]
        tunnel: w571 -> [w640]
        tunnel: w570 -> [w639]
        tunnel: w569 -> [w638]
        tunnel: w568 -> [w637]
        tunnel: [w636] -> w451
        tunnel: [w635] -> w450
        tunnel: [w634] -> w449
        tunnel: [w633] -> w448
        tunnel: [w632] -> w447
        tunnel: [w631] -> w422
        tunnel: [w630] -> w421
        tunnel: [w629] -> w419
        tunnel: [w628] -> w418
        tunnel: [w627] -> w417
        frame #0 {
          n165 = call-poly <vilib>:"DAQmx Write.vi"("task/channels in"=w600, "data"=w593, "error in"=w603) -> ("task out"=w601:refnum<k21>, "error out"=w602:errorcluster)  [unwired: 10 in, 1 out]
          n166 = call-poly <vilib>:"DAQmx Write.vi"("task/channels in"=w598, "data"=w594, "error in"=w599) -> ("task out"=w597:refnum<k21>, "error out"=w596:errorcluster)  [unwired: 10 in, 1 out]
        }
        frame #1 {
          n167 = call-poly <vilib>:"DAQmx Write.vi"("task/channels in"=w616, "data"=w612, "error in"=w613) -> ("task out"=w615:refnum<k21>, "error out"=w614:errorcluster)  [unwired: 10 in, 1 out]
        }
        frame #2 {
          n168 = call <vilib>:"DAQmx Start Task.vi"("task/channels in"=w646, "error in"=w644) -> ("task out"=w636:refnum<k21>, "error out"=w631:errorcluster)  [unwired: 12 in]
          n169 = call <vilib>:"DAQmx Start Task.vi"("task/channels in"=w645, "error in"=w643) -> ("task out"=w635:refnum<k21>, "error out"=w630:errorcluster)  [unwired: 12 in]
          n170 = call <vilib>:"DAQmx Start Task.vi"("task/channels in"=w642, "error in"=w639) -> ("task out"=w634:refnum<k21>, "error out"=w629:errorcluster)  [unwired: 12 in]
          n171 = call <vilib>:"DAQmx Start Task.vi"("task/channels in"=w641, "error in"=w638) -> ("task out"=w633:refnum<k21>, "error out"=w628:errorcluster)  [unwired: 12 in]
          n172 = call <vilib>:"DAQmx Start Task.vi"("task/channels in"=w640, "error in"=w637) -> ("task out"=w632:refnum<k21>, "error out"=w627:errorcluster)  [unwired: 12 in]
        }
      }
      n173 = call <vilib>:"DAQmx Start Task.vi"("task/channels in"=w565, "error in"=w564) -> ("task out"=w544:refnum<k21>, "error out"=w423:errorcluster)  [unwired: 12 in]
      n174 = Build Array(w544, w451, w450) -> (w543:refnum<k21>[])
      n175 = Merge Errors(w423, w422, w421, w419, w418, w417, w414) -> (w420:errorcluster)
      n176 = Build Array(w449, w448, w447) -> (w446:refnum<k21>[])
    }
    frame 2 {
      w675 = tag "PXI_Clk10" ("RefClk.Src")
      w662 = 10123 items=["Finite Samples"=10178, "Continuous Samples"=10123] ("sample mode")
      # "master AI last"
      # "MASTER"
      n177 = Index Array(array=w739) -> (element #1=w764:T4, element #2=w726:T4)  [unwired: 2 in]
      n178 = Index Array(array=w714) -> (element #1=w713:T5, element #2=w692:T5)  [unwired: 2 in]
      n179 = Unbundle By Name(w764) -> ("AI.Min"=w737:dbl, "AI.Max"=w738:dbl, "Input physical channels"=w749:tag, "AI.Coupling"=w736:i32)
      n180 = Unbundle By Name(w726) -> ("AI.Min"=w733:dbl, "AI.Max"=w732:dbl, "Input physical channels"=w727:tag, "AI.Coupling"=w734:i32)
      n181 = Unbundle By Name(w713) -> ("AO.Min"=w710:dbl, "AO. Max"=w711:dbl, "Output physical channels"=w712:tag)
      n182 = Unbundle By Name(w692) -> ("AO.Min"=w695:dbl, "AO. Max"=w694:dbl, "Output physical channels"=w693:tag)
      n183 = call-poly <vilib>:"DAQmx Create Virtual Channel.vi"("maximum value"=w738, "minimum value"=w737, "input terminal configuration"=w649, "physical channels"=w749, "error in"=w654) -> ("task out"=w748:refnum<k21>, "error out"=w747:errorcluster)  [unwired: 9 in]
      n184 = call-poly <vilib>:"DAQmx Create Virtual Channel.vi"("maximum value"=w732, "minimum value"=w733, "input terminal configuration"=w649, "physical channels"=w727, "error in"=w654) -> ("task out"=w728:refnum<k21>, "error out"=w729:errorcluster)  [unwired: 9 in]
      n185 = call-poly <vilib>:"DAQmx Create Virtual Channel.vi"("maximum value"=w711, "minimum value"=w710, "output terminal configuration"=w650, "physical channels"=w712, "error in"=w654) -> ("task out"=w674:refnum<k21>, "error out"=w673:errorcluster)  [unwired: 9 in]
      n186 = call-poly <vilib>:"DAQmx Create Virtual Channel.vi"("maximum value"=w694, "minimum value"=w695, "output terminal configuration"=w650, "physical channels"=w693, "error in"=w654) -> ("task out"=w696:refnum<k21>, "error out"=w697:errorcluster)  [unwired: 9 in]
      n187 = Unbundle By Name(w664) -> ("#s"=w661:dbl, "Fs"=w663:dbl)
      n188 = property class="DAQmx Channel"(reference=w748, error in=w747, "AI.Coupling"=w736) -> (reference out=w746:refnum<k21>, error out=w745:errorcluster)
      n189 = property class="DAQmx Channel"(reference=w728, error in=w729, "AI.Coupling"=w734) -> (reference out=w730:refnum<k21>, error out=w731:errorcluster)
      n190 = Multiply(x=w742, y=w661) -> (x*y=w666:dbl)
      n191 = call <vilib>:"DAQmx Configure Input Buffer.vi"("task/channels in"=w746, "buffer size (in samples per channel)"=w666, "error in"=w745) -> ("task out"=w744:refnum<k21>, "error out"=w743:errorcluster)  [unwired: 11 in]
      n192 = call <vilib>:"DAQmx Configure Input Buffer.vi"("task/channels in"=w730, "buffer size (in samples per channel)"=w666, "error in"=w731) -> ("task out"=w725:refnum<k21>, "error out"=w724:errorcluster)  [unwired: 11 in]
      n193 = call-poly <vilib>:"DAQmx Timing.vi"("task/channels in"=w696, "sample mode"=w662, "samples per channel"=w661, "rate"=w663, "error in"=w697) -> ("task out"=w699:refnum<k21>, "error out"=w700:errorcluster)  [unwired: 9 in]
      n194 = call-poly <vilib>:"DAQmx Timing.vi"("task/channels in"=w744, "sample mode"=w662, "samples per channel"=w661, "rate"=w663, "error in"=w743) -> ("task out"=w763:refnum<k21>, "error out"=w735:errorcluster)  [unwired: 9 in]
      n195 = call-poly <vilib>:"DAQmx Timing.vi"("task/channels in"=w725, "sample mode"=w662, "samples per channel"=w661, "rate"=w663, "error in"=w724) -> ("task out"=w723:refnum<k21>, "error out"=w722:errorcluster)  [unwired: 9 in]
      n196 = call-poly <vilib>:"DAQmx Timing.vi"("task/channels in"=w674, "sample mode"=w662, "samples per channel"=w661, "rate"=w663, "error in"=w673) -> ("task out"=w708:refnum<k21>, "error out"=w707:errorcluster)  [unwired: 9 in]
      n197 = property class="DAQmx Timing" props=["More:Reference Clock:Source", "SampQuant.SampPerChan", "SampClk.Timebase.Rate", "SampClk.Timebase.Src"](reference=w763, error in=w735, "More:Reference Clock:Source"=w675) -> (reference out=w679:refnum<k21>, error out=w678:errorcluster, "SampQuant.SampPerChan"=w652:dbl, "SampClk.Timebase.Rate"=w651:dbl)  [unwired: 1 out]
      n198 = call "Get Terminal Name with Device Prefix.vi"("error in (no error)"=w678, "Local Terminal Name"="SyncPulse", "task/channels in"=w679) -> ("error out"=w758:errorcluster, "Terminal Name with Device Prefix"=w676:tag, "task out"=w759:refnum<k21>)  [unwired: 6 in]
      n199 = property class="DAQmx Timing"(reference=w723, error in=w722, "More:Reference Clock:Source"=w675, "More:Synchronization Pulse:Source"=w676) -> (reference out=w721:refnum<k21>, error out=w720:errorcluster)
      n200 = property class="DAQmx Timing"(reference=w708, error in=w707, "More:Reference Clock:Source"=w675, "More:Synchronization Pulse:Source"=w676) -> (reference out=w709:refnum<k21>, error out=w706:errorcluster)
      n201 = property class="DAQmx Timing"(reference=w699, error in=w700, "More:Reference Clock:Source"=w675, "More:Synchronization Pulse:Source"=w676) -> (reference out=w698:refnum<k21>, error out=w701:errorcluster)
      n202 = local write "SampQuant.SampPerChan"(w652) -> ()
      n203 = local write "SampClk.Timebase.Rate"(w651) -> ()
      n204 = call "Get Terminal Name with Device Prefix.vi"("error in (no error)"=w758, "Local Terminal Name"="ai/StartTrigger", "task/channels in"=w759) -> ("error out"=w756:errorcluster, "Terminal Name with Device Prefix"=w689:tag, "task out"=w757:refnum<k21>)  [unwired: 6 in]
      n205 = call-poly <vilib>:"DAQmx Trigger.vi"("task/channels in"=w721, "source"=w689, "error in"=w720) -> ("task out"=w719:refnum<k21>, "error out"=w718:errorcluster)  [unwired: 11 in]
      n206 = call-poly <vilib>:"DAQmx Trigger.vi"("task/channels in"=w709, "source"=w689, "error in"=w706) -> ("task out"=w705:refnum<k21>, "error out"=w704:errorcluster)  [unwired: 11 in]
      n207 = call-poly <vilib>:"DAQmx Trigger.vi"("task/channels in"=w698, "source"=w689, "error in"=w701) -> ("task out"=w702:refnum<k21>, "error out"=w703:errorcluster)  [unwired: 11 in]
      n208 = property class="DAQmx Timing"(reference=w757, error in=w756) -> (reference out=w753:refnum<k21>, error out=w754:errorcluster, "SyncPulse.SyncTime"=w755:dbl)
      n209 = property class="DAQmx Timing"(reference=w719, error in=w718) -> (reference out=w715:refnum<k21>, error out=w688:errorcluster, "SyncPulse.SyncTime"=w716:dbl)
      n210 = property class="DAQmx Timing"(reference=w705, error in=w704) -> (reference out=w687:refnum<k21>, error out=w685:errorcluster, "SyncPulse.SyncTime"=w691:dbl)
      n211 = property class="DAQmx Timing"(reference=w702, error in=w703) -> (reference out=w686:refnum<k21>, error out=w684:errorcluster, "SyncPulse.SyncTime"=w690:dbl)
      n212 = Build Array(w755, w716, w691, w690) -> (w752:dbl[])
      n213 = Array Max & Min(array=w752) -> (max value=w717:dbl)  [unwired: 3 out]
      n214 = property class="DAQmx Timing"(reference=w753, error in=w754, "SyncPulse.MinDelayToStart"=w717) -> (reference out=w750:refnum<k21>, error out=w751:errorcluster)
      n215 = call "4461 - Create AO waveforms.vi"("error in (no error)"=w654, "sampling info"=w664, "AO"=w665) -> ("error out"=w653:errorcluster, "AO Array"=w655:waveform(dbl)[])  [unwired: 5 in, 2 out]
      n216 = Index Array(array=w655) -> (element #1=w667:waveform(dbl), element #2=w672:waveform(dbl), element #3=w671:waveform(dbl), element #4=w670:waveform(dbl))  [unwired: 4 in]
      n217 = Build Array(w667, w672) -> (w669:waveform(dbl)[])
      n218 = Build Array(w671, w670) -> (w668:waveform(dbl)[])
      n219 = flat-sequence {
        tunnel: w751 -> [w792]
        tunnel: w750 -> [w793]
        tunnel: [w793] -> w781
        tunnel: [w792] -> w780
        tunnel: [w791] -> w779
        tunnel: w715 -> [w791]
        tunnel: [w790] -> w778
        tunnel: w688 -> [w790]
        tunnel: [w789] -> w777
        tunnel: w687 -> [w789]
        tunnel: [w785] -> w776
        tunnel: w686 -> [w786]
        tunnel: [w788] -> w775
        tunnel: w685 -> [w788]
        tunnel: w684 -> [w787]
        tunnel: [w784] -> w774
        tunnel: [w783] -> w773
        tunnel: w669 -> [w783]
        tunnel: w668 -> [w782]
        tunnel: [w804] -> w772
        tunnel: [w803] -> w771
        tunnel: w781 -> [w804]
        tunnel: w780 -> [w803]
        tunnel: [w802] -> w770
        tunnel: w779 -> [w802]
        tunnel: [w801] -> w769
        tunnel: w778 -> [w801]
        tunnel: [w797] -> w768
        tunnel: w777 -> [w798]
        tunnel: [w800] -> w767
        tunnel: w776 -> [w800]
        tunnel: [w796] -> w766
        tunnel: w775 -> [w795]
        tunnel: [w799] -> w765
        tunnel: w774 -> [w799]
        tunnel: w773 -> [w794]
        tunnel: [w818] -> w762
        tunnel: [w817] -> w761
        tunnel: w772 -> [w818]
        tunnel: w771 -> [w817]
        tunnel: w770 -> [w816]
        tunnel: w769 -> [w815]
        tunnel: w768 -> [w814]
        tunnel: w767 -> [w813]
        tunnel: w766 -> [w812]
        tunnel: w765 -> [w811]
        tunnel: [w810] -> w683
        tunnel: [w809] -> w682
        tunnel: [w808] -> w681
        tunnel: [w807] -> w659
        tunnel: [w806] -> w657
        tunnel: [w805] -> w656
        frame #0 {
          n220 = call-poly <vilib>:"DAQmx Write.vi"("task/channels in"=w786, "data"=w782, "error in"=w787) -> ("task out"=w785:refnum<k21>, "error out"=w784:errorcluster)  [unwired: 10 in, 1 out]
        }
        frame #1 {
          n221 = call-poly <vilib>:"DAQmx Write.vi"("task/channels in"=w798, "data"=w794, "error in"=w795) -> ("task out"=w797:refnum<k21>, "error out"=w796:errorcluster)  [unwired: 10 in, 1 out]
        }
        frame #2 {
          n222 = call <vilib>:"DAQmx Start Task.vi"("task/channels in"=w816, "error in"=w815) -> ("task out"=w810:refnum<k21>, "error out"=w807:errorcluster)  [unwired: 12 in]
          n223 = call <vilib>:"DAQmx Start Task.vi"("task/channels in"=w814, "error in"=w812) -> ("task out"=w809:refnum<k21>, "error out"=w806:errorcluster)  [unwired: 12 in]
          n224 = call <vilib>:"DAQmx Start Task.vi"("task/channels in"=w813, "error in"=w811) -> ("task out"=w808:refnum<k21>, "error out"=w805:errorcluster)  [unwired: 12 in]
        }
      }
      n225 = call <vilib>:"DAQmx Start Task.vi"("task/channels in"=w762, "error in"=w761) -> ("task out"=w741:refnum<k21>, "error out"=w660:errorcluster)  [unwired: 12 in]
      n226 = Build Array(w741, w683) -> (w740:refnum<k21>[])
      n227 = Merge Errors(w660, w659, w657, w656, w653) -> (w658:errorcluster)
      n228 = Build Array(w682, w681) -> (w680:refnum<k21>[])
    }
    frame 1 {
      w840 = tag "PXI_Clk10" ("RefClk.Src")
      w830 = 10123 items=["Finite Samples"=10178, "Continuous Samples"=10123] ("sample mode")
      # "master AI last"
      # "MASTER"
      n229 = Index Array(array=w867) -> (element=w892:T4)  [unwired: 1 in]
      n230 = Index Array(array=w861) -> (element=w860:T5)  [unwired: 1 in]
      n231 = Unbundle By Name(w892) -> ("AI.Min"=w865:dbl, "AI.Max"=w866:dbl, "Input physical channels"=w877:tag, "AI.Coupling"=w864:i32)
      n232 = Unbundle By Name(w860) -> ("AO.Min"=w857:dbl, "AO. Max"=w858:dbl, "Output physical channels"=w859:tag)
      n233 = call-poly <vilib>:"DAQmx Create Virtual Channel.vi"("maximum value"=w866, "minimum value"=w865, "input terminal configuration"=w820, "physical channels"=w877, "error in"=w824) -> ("task out"=w876:refnum<k21>, "error out"=w875:errorcluster)  [unwired: 9 in]
      n234 = call-poly <vilib>:"DAQmx Create Virtual Channel.vi"("maximum value"=w858, "minimum value"=w857, "output terminal configuration"=w819, "physical channels"=w859, "error in"=w824) -> ("task out"=w839:refnum<k21>, "error out"=w838:errorcluster)  [unwired: 9 in]
      n235 = Unbundle By Name(w832) -> ("#s"=w829:dbl, "Fs"=w831:dbl)
      n236 = property class="DAQmx Channel"(reference=w876, error in=w875, "AI.Coupling"=w864) -> (reference out=w874:refnum<k21>, error out=w873:errorcluster)
      n237 = Multiply(x=w870, y=w829) -> (x*y=w834:dbl)
      n238 = call <vilib>:"DAQmx Configure Input Buffer.vi"("task/channels in"=w874, "buffer size (in samples per channel)"=w834, "error in"=w873) -> ("task out"=w872:refnum<k21>, "error out"=w871:errorcluster)  [unwired: 11 in]
      n239 = call-poly <vilib>:"DAQmx Timing.vi"("task/channels in"=w872, "sample mode"=w830, "samples per channel"=w829, "rate"=w831, "error in"=w871) -> ("task out"=w891:refnum<k21>, "error out"=w863:errorcluster)  [unwired: 9 in]
      n240 = call-poly <vilib>:"DAQmx Timing.vi"("task/channels in"=w839, "sample mode"=w830, "samples per channel"=w829, "rate"=w831, "error in"=w838) -> ("task out"=w855:refnum<k21>, "error out"=w854:errorcluster)  [unwired: 9 in]
      n241 = property class="DAQmx Timing" props=["More:Reference Clock:Source", "SampQuant.SampPerChan", "SampClk.Timebase.Rate", "SampClk.Timebase.Src"](reference=w891, error in=w863, "More:Reference Clock:Source"=w840) -> (reference out=w844:refnum<k21>, error out=w843:errorcluster, "SampQuant.SampPerChan"=w822:dbl, "SampClk.Timebase.Rate"=w821:dbl)  [unwired: 1 out]
      n242 = call "Get Terminal Name with Device Prefix.vi"("error in (no error)"=w843, "Local Terminal Name"="SyncPulse", "task/channels in"=w844) -> ("error out"=w886:errorcluster, "Terminal Name with Device Prefix"=w841:tag, "task out"=w887:refnum<k21>)  [unwired: 6 in]
      n243 = property class="DAQmx Timing"(reference=w855, error in=w854, "More:Reference Clock:Source"=w840, "More:Synchronization Pulse:Source"=w841) -> (reference out=w856:refnum<k21>, error out=w853:errorcluster)
      n244 = local write "SampQuant.SampPerChan"(w822) -> ()
      n245 = local write "SampClk.Timebase.Rate"(w821) -> ()
      n246 = call "Get Terminal Name with Device Prefix.vi"("error in (no error)"=w886, "Local Terminal Name"="ai/StartTrigger", "task/channels in"=w887) -> ("error out"=w884:errorcluster, "Terminal Name with Device Prefix"=w849:tag, "task out"=w885:refnum<k21>)  [unwired: 6 in]
      n247 = call-poly <vilib>:"DAQmx Trigger.vi"("task/channels in"=w856, "source"=w849, "error in"=w853) -> ("task out"=w852:refnum<k21>, "error out"=w851:errorcluster)  [unwired: 11 in]
      n248 = property class="DAQmx Timing"(reference=w885, error in=w884) -> (reference out=w881:refnum<k21>, error out=w882:errorcluster, "SyncPulse.SyncTime"=w883:dbl)
      n249 = property class="DAQmx Timing"(reference=w852, error in=w851) -> (reference out=w848:refnum<k21>, error out=w847:errorcluster, "SyncPulse.SyncTime"=w850:dbl)
      n250 = Build Array(w883, w850) -> (w880:dbl[])
      n251 = Array Max & Min(array=w880) -> (max value=w862:dbl)  [unwired: 3 out]
      n252 = property class="DAQmx Timing"(reference=w881, error in=w882, "SyncPulse.MinDelayToStart"=w862) -> (reference out=w878:refnum<k21>, error out=w879:errorcluster)
      n253 = call "4461 - Create AO waveforms.vi"("error in (no error)"=w824, "sampling info"=w832, "AO"=w833) -> ("error out"=w823:errorcluster, "AO Array"=w825:waveform(dbl)[])  [unwired: 5 in, 2 out]
      n254 = Index Array(array=w825) -> (element #1=w835:waveform(dbl), element #2=w837:waveform(dbl))  [unwired: 2 in]
      n255 = Build Array(w835, w837) -> (w836:waveform(dbl)[])
      n256 = flat-sequence {
        tunnel: w879 -> [w905]
        tunnel: w878 -> [w906]
        tunnel: [w906] -> w901
        tunnel: [w905] -> w900
        tunnel: [w904] -> w899
        tunnel: w848 -> [w904]
        tunnel: [w903] -> w898
        tunnel: w847 -> [w903]
        tunnel: [w902] -> w897
        tunnel: w836 -> [w902]
        tunnel: [w913] -> w896
        tunnel: [w912] -> w895
        tunnel: w901 -> [w913]
        tunnel: w900 -> [w912]
        tunnel: [w910] -> w894
        tunnel: w899 -> [w911]
        tunnel: [w909] -> w893
        tunnel: w898 -> [w908]
        tunnel: w897 -> [w907]
        tunnel: [w919] -> w890
        tunnel: [w918] -> w889
        tunnel: w896 -> [w919]
        tunnel: w895 -> [w918]
        tunnel: w894 -> [w917]
        tunnel: w893 -> [w916]
        tunnel: [w915] -> w846
        tunnel: [w914] -> w826
        frame #0 {
        }
        frame #1 {
          n257 = call-poly <vilib>:"DAQmx Write.vi"("task/channels in"=w911, "data"=w907, "error in"=w908) -> ("task out"=w910:refnum<k21>, "error out"=w909:errorcluster)  [unwired: 10 in, 1 out]
        }
        frame #2 {
          n258 = call <vilib>:"DAQmx Start Task.vi"("task/channels in"=w917, "error in"=w916) -> ("task out"=w915:refnum<k21>, "error out"=w914:errorcluster)  [unwired: 12 in]
        }
      }
      n259 = call <vilib>:"DAQmx Start Task.vi"("task/channels in"=w890, "error in"=w889) -> ("task out"=w869:refnum<k21>, "error out"=w828:errorcluster)  [unwired: 12 in]
      n260 = Build Array(w869) -> (w868:refnum<k21>[])
      n261 = Merge Errors(w828, w826, w823) -> (w827:errorcluster)
      n262 = Build Array(w846) -> (w845:refnum<k21>[])
    }
  }
  "AI task" <- w14
  "AO Task" <- w12
  "error out" <- w6
  n263 = Initialize Array(0.0 ("element"), 8 ("dimension size")) -> (→"phase log":dbl[])
